vi "chaos crest connect.vi"(11 "handleConnection":u32) -> (3 "nok":i32)   [LabVIEW 2014, in "libcommon-crest.lvlib"]
doc: "int chaos_crest_connect(chaos_crest_handle_t h);"
uses:
  libcommon-crest.lvlib
  chaos-i686-dynamic-release/lib/libcommon-crest.so
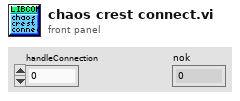
[diagram p1: front panel]
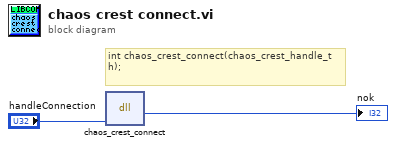
[diagram p0: block diagram]
diagram:
  # "int chaos_crest_connect(chaos_crest_handle_t h);"
  n1 = dll-call lib="home/chaos/chaos_bundle/chaos-i686-dynamic-release/lib/libcommon-crest.*" fn="chaos_crest_connect"("handleConnection"="handleConnection") -> (→"nok":i32)  [unwired: 4 in, 2 out]
